vi "Text control 2 v0.4.vi"() -> ()   [LabVIEW 2016]
panel:
  out "Ion vs time":cluster{"Y data in":dbl[], "X data in":dbl[]}[](graph)
  out "Ig":dbl format="%.2e"
  out "Id":dbl format="%.2e"
  out "Is":dbl format="%.2e"
  out "I vs Vg":cluster{"Y data in":dbl[], "X data in":dbl[]}[](graph)
  in  "Suffix":string=".txt"
  in  "Prefix":string="-transfer-"
  in  "Panel Controls 2":T1={"Emergency Stop"=refnum, "TransGraph Max"=1e-05, "Text/Graph (text=false)"=TRUE, "TransGraph Min"=1e-11} {"TransGraph Min" format="%.2e"; "TransGraph Max" format="%.2e"}
  out "Currently running:":string="#output s 0 0 0 -0.008 0.008 0.002"
  in  "Lines left to run:":string
  in  "Standby":T2
  in  "Full Reset":bool
  in  "SMU4":cluster{"on/off":bool, "Voltage":dbl} {"Voltage" min=-100.0 max=100.0 format="%.2f"}
  in  "Source/Drain Range":u8(slide)=6 max=11 scale=0.0..11.0
  in  "Source/Drain\nRange mode":u16(ring) items=["Auto", "Limited", "Fixed"]
  in  "Gate Range":u8(slide)=6 max=11 scale=0.0..11.0
  in  "Gate Range\nmode":u16(ring) items=["Auto", "Limited", "Fixed"]
  in  "Gate":T3={"Gate Start"=0.0, "Gate Stop"=2.0, "Gate Step (linear only)"=1.0, "Gate Compliance"=0.0001, "Gate PComp"=0.0, "Range mode"=0, "Range"=6} {"Range" max=11 scale=0.0..11.0; "Range mode" items=["Auto", "Limited", "Fixed"]; "Gate PComp" format="%^.2e"; "Gate Compliance" format="%^.2e"; "Gate Step (linear only)" format="%^.4e"; "Gate Stop" format="%^.4e"; "Gate Start" format="%^.4e"}
  in  "Drain 2":T4={"Drain Start"=0.0, "Drain Stop"=2.0, "Drain Compliance"=0.0001, "Drain Step"=1.0, "Drain PComp"=0.0, "Range mode"=0, "Range"=6} {"Range" max=11 scale=0.0..11.0; "Range mode" items=["Auto", "Limited", "Fixed"]; "Drain PComp" format="%^.2e"; "Drain Step" format="%^.4e"; "Drain Compliance" format="%^.2e"; "Drain Stop" format="%^.4e"; "Drain Start" format="%^.4e"}
  in  "Timings 2":T5={"integration time"=0, "Short/Long integration time"=0.00064, "hold time (sec)"=0.0, "delay time (sec)"=0.0, "Step Time (0 disables)"=0.0, "sweep method"=0, "Pulse period"=0.005, "Base voltage"=0.0, "Pulse width"=0.0005} {"Pulse width" min=0.0005 max=0.1 step=0.0001 format="%.4f"; "Base voltage" format="%^.4e"; "Pulse period" min=0.005 max=1.0 step=0.0001 format="%.4f"; "sweep method" items=["Continuous", "Pulsed"]; "Step Time (0 disables)" format="%.2f"; "delay time (sec)" format="%.4f"; "hold time (sec)" format="%.4f"; "Short/Long integration time" format="%^.0e"; "integration time" scale=0.0..2.0}
  in  "Panel Controls":T6={"Emergency Stop"=refnum, "TransGraph Max"=1e-05, "Text/Graph (text=false)"=TRUE} {"TransGraph Max" format="%.2e"}
  in  "Interrupt run":bool
  in  "Drain: Compliance":dbl=0.001 format="%.8f"
  in  "Gate: Compliance":dbl=0.001 format="%.8f"
  out "Path":path=path "C:/users/rlp38/09Apr2009LTtesting/test2.txt"
  in  "hold time /s":dbl format="%.2f"
  in  "delay time /s":dbl format="%.2f"
  in  "integration time":u32(slide) max=2 step=1 scale=0.0..2.0
  in  "Integration time (short)":dbl=0.0019 min=8e-05 max=0.0019 step=8e-05 format="%^.0e"
  in  "Integration time (long)":dbl=0.32 min=0.04 max=2.0 step=0.02 format="%.2f"
  in  "Step delay /s":dbl format="%.2f"
  in  "Program":string="#pulsedstressV d 0.03 20 0 0.5 0.0827 5\n#\n#itime m\n#gaterangemode a\n#drainrangemode a\n#pulsed on 0.05 0 0.02\n#transfer d -10 40 1 5 40 35\n#transfer d -10 40 1 5 40 35\n#transfer d -10 40 1 5 40 35\n#output d 0 40 20 0 40 1\n#\n#\n#sample 1 0.008 221 6 0.003\n#samplei 400e-6 200 6 0.002 0.1\n#vsu2pulse -10 4\n#\n#stressV 0.016 0.03 2e-4 0.1e-3 11\n#stressI 220e-7 0.08 15\n#transfer s -1 1 0.5 -0.005 0.005 0.005\n#output s 0 0 0 -0.008 0.008 0.002\n"
  # "Syntax:\nitime [s|m|l]\ngaterangemode [a|l|f]\ndrainrangemode [a|l|f]\npulsed [on|off] PulsePeriod(sec) PulseBaseVoltage PulseONWidth(sec)\nstandby [on l off]\nwait NumMilliseconds\nwait-min NumMinutes\n# texthere = comment\ntransfer [s|d] VgStart VgStop VgStep VdStart VdStop VdStep\noutput [s|d] VgStart VgStop VgStep VdStart VdStop VdStep\nsample Vg Vd NumSamples Time(s) SampleInterval(s)\nsamplei Idg NumSamples Time(s) SampleInterval(s) VDGcompliance\n# if in doubt use SampleInterval(s) = 0.004\nstressV VG VD IGcompliance IDcompliance Duration(sec)\nstressI IDG VDGcompliance Duration(sec)\nvsu2pulse Bias Duration(s)\npulsedstressV [s|d] VEstop VgON VgOFF Period(s) PulseONwidth(s) Vd\nsample-fpp Vg Vd NumSamples Time\nresample-fpp Vg Vd\ntransfer-fpp [s|d] VgStart VgStop VgStep VdStart VdStop VdStep\noutput-fpp [s|d] VgStart VgStop VgStep VdStart VdStop VdStep"
  # "Original Filename (.txt is removed)-Prefix-ElapsedTime (in sec)-Suffix (must include .txt)"
  # "100 samples is approx 13s with medium integration"
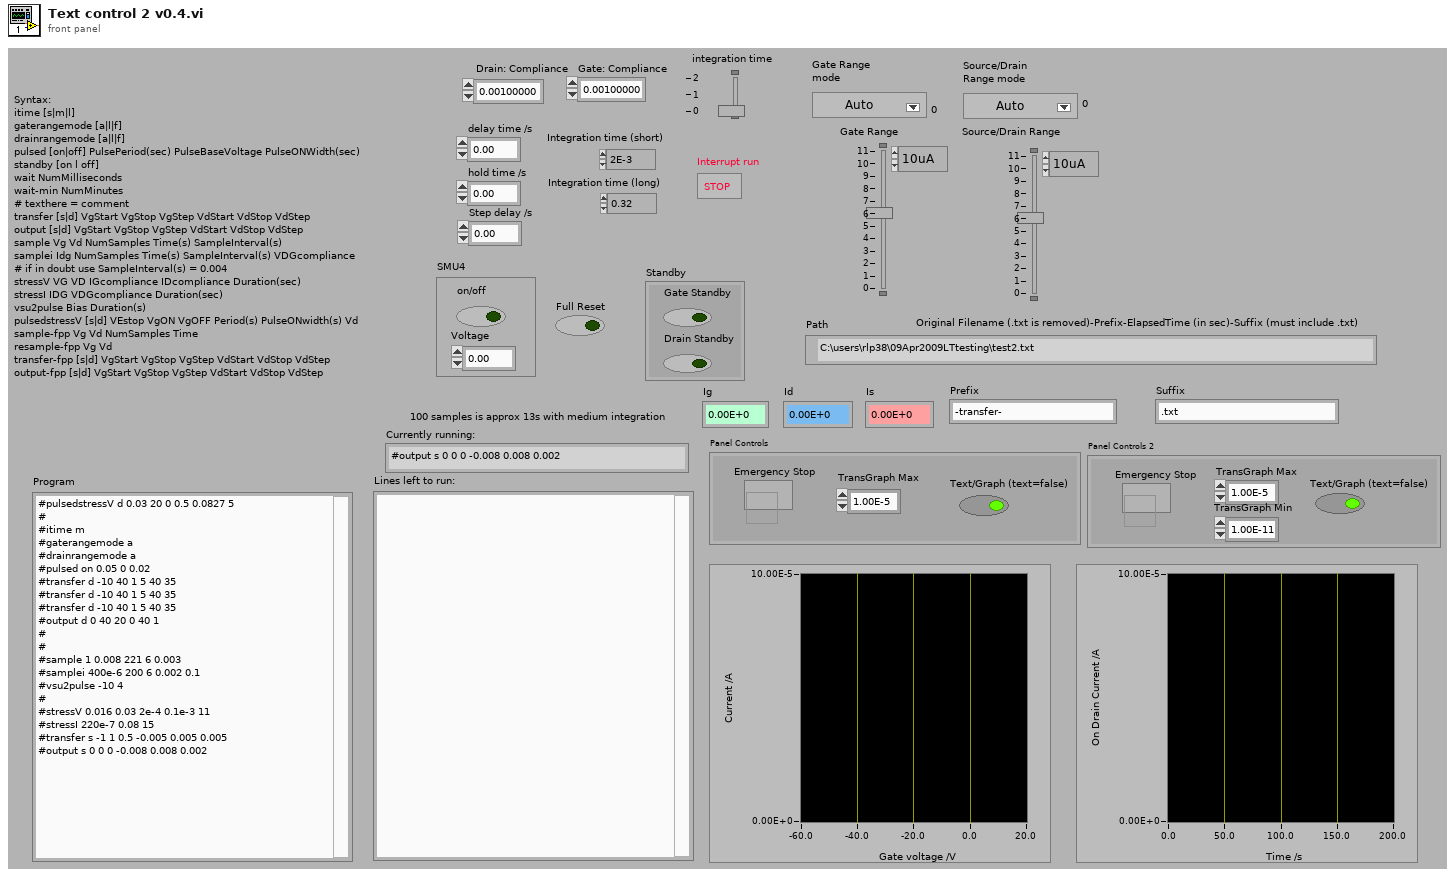
[diagram p1: front panel]
types:
  T1 = cluster{"Emergency Stop":refnum<vi>, "TransGraph Max":dbl, "Text/Graph (text=false)":bool, "TransGraph Min":dbl}
  T2 = cluster{"Gate Standby":bool, "Drain Standby":bool}
  T3 = cluster{"Gate Start":dbl, "Gate Stop":dbl, "Gate Step (linear only)":dbl, "Gate Compliance":dbl, "Gate PComp":dbl, "Range mode":u16, "Range":u8}
  T4 = cluster{"Drain Start":dbl, "Drain Stop":dbl, "Drain Compliance":dbl, "Drain Step":dbl, "Drain PComp":dbl, "Range mode":u16, "Range":u8}
  T5 = cluster{"integration time":u32, "Short/Long integration time":dbl, "hold time (sec)":dbl, "delay time (sec)":dbl, "Step Time (0 disables)":dbl, "sweep method":u16, "Pulse period":dbl, "Base voltage":dbl, "Pulse width":dbl}
  T6 = cluster{"Emergency Stop":refnum<vi>, "TransGraph Max":dbl, "Text/Graph (text=false)":bool}
  T7 = enum16{"open", "replace", "create", "open or create", "replace or create", "replace or create with confirmation"}
  T8 = cluster{"V2 Start":dbl, "V2 Step":dbl, "Number of points":i32}
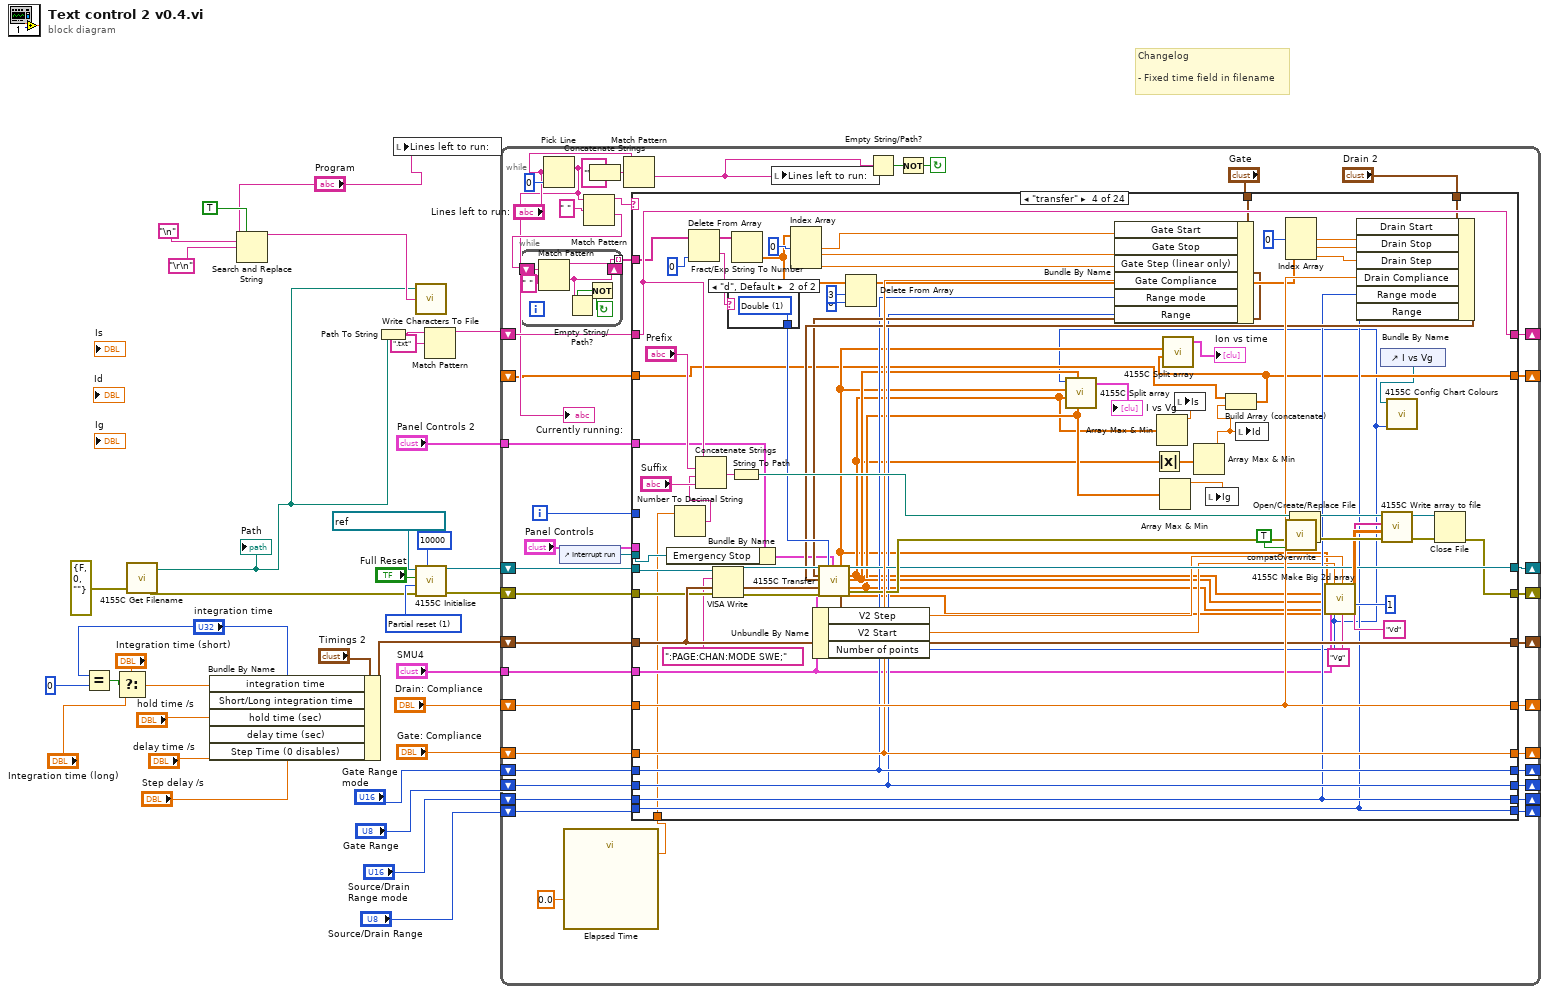
[diagram p0: block diagram]
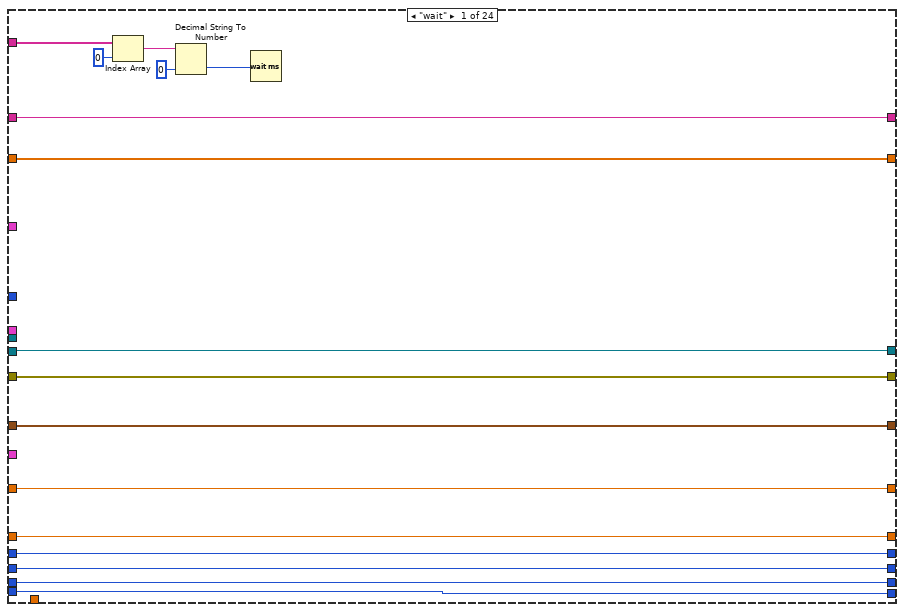
[diagram p2: hidden frame]
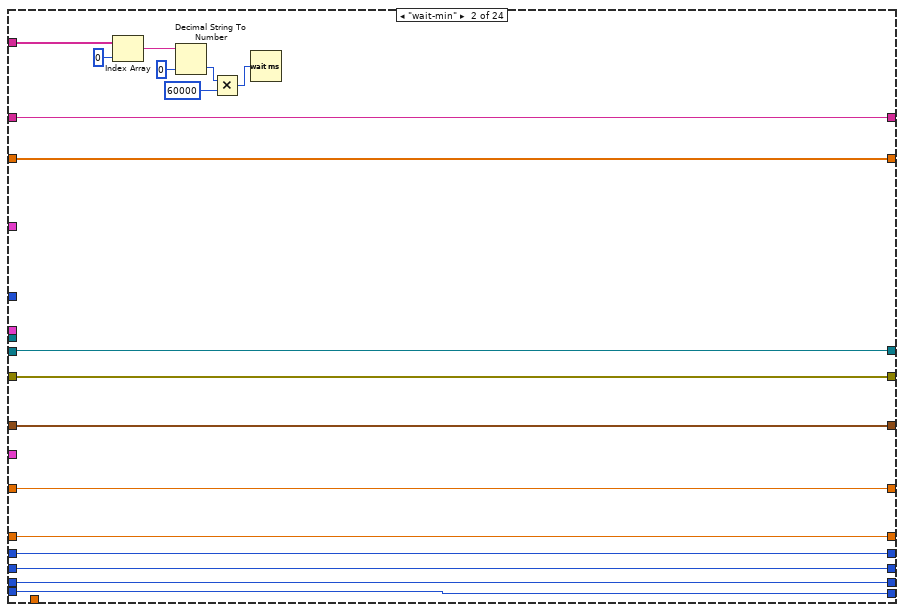
[diagram p3: hidden frame]
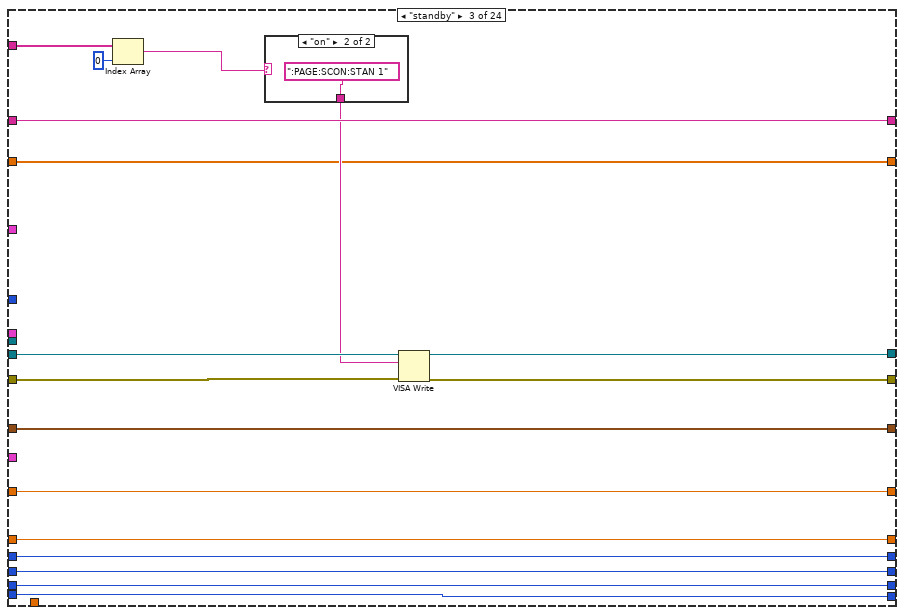
[diagram p4: hidden frame]
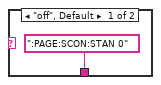
[diagram p5: hidden frame]
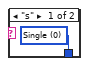
[diagram p6: hidden frame]
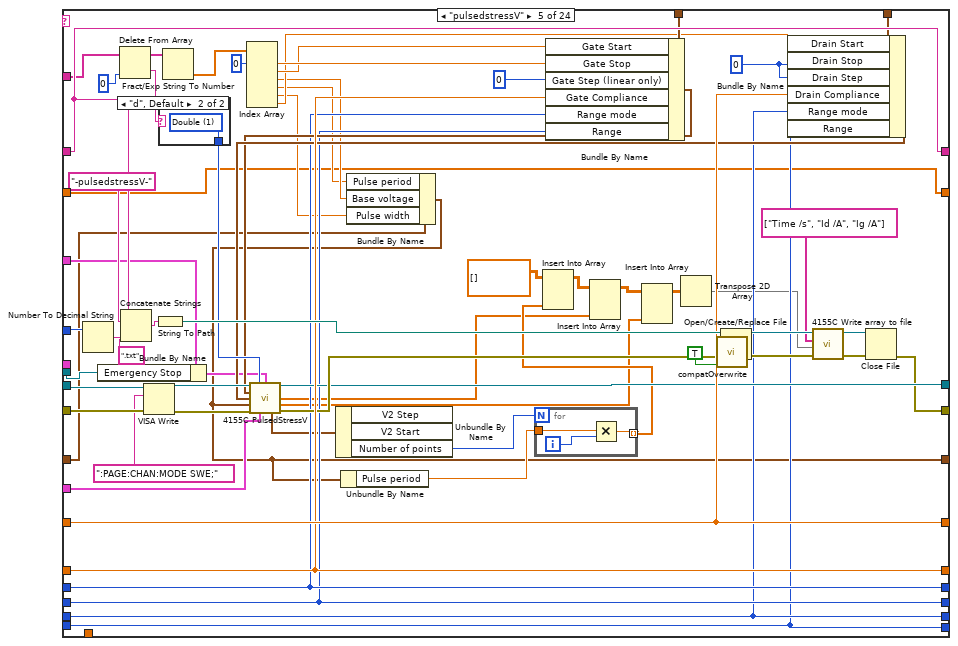
[diagram p7: hidden frame]
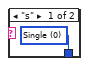
[diagram p8: hidden frame]
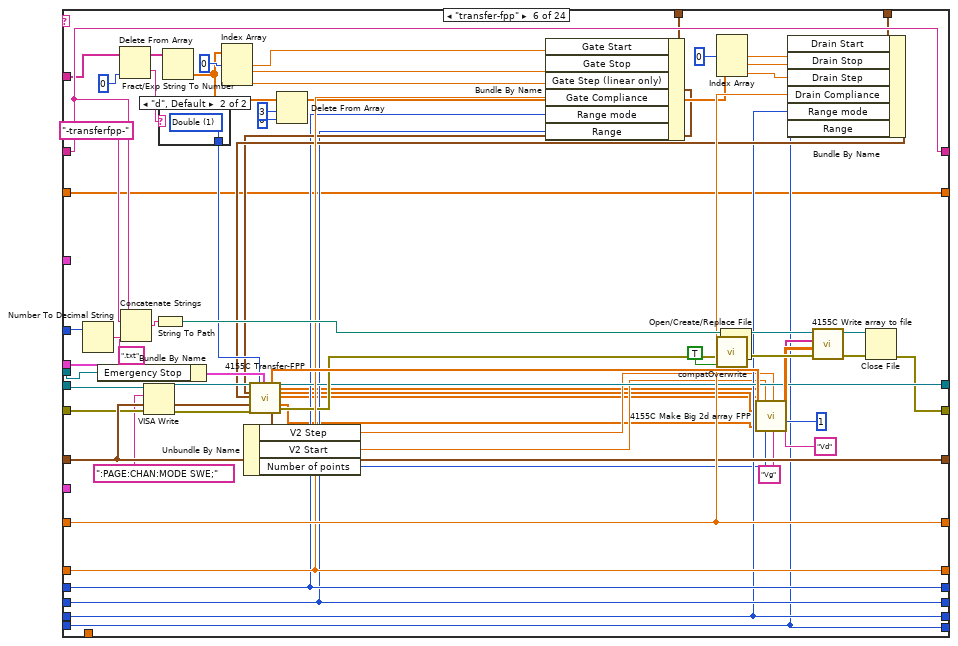
[diagram p9: hidden frame]
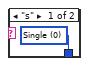
[diagram p10: hidden frame]
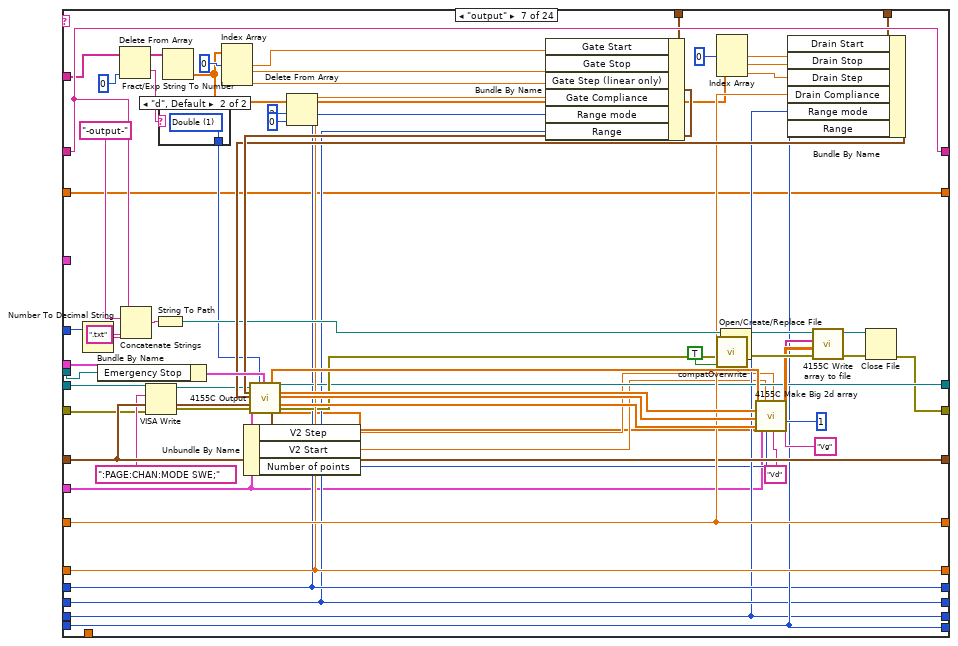
[diagram p11: hidden frame]
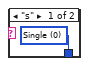
[diagram p12: hidden frame]
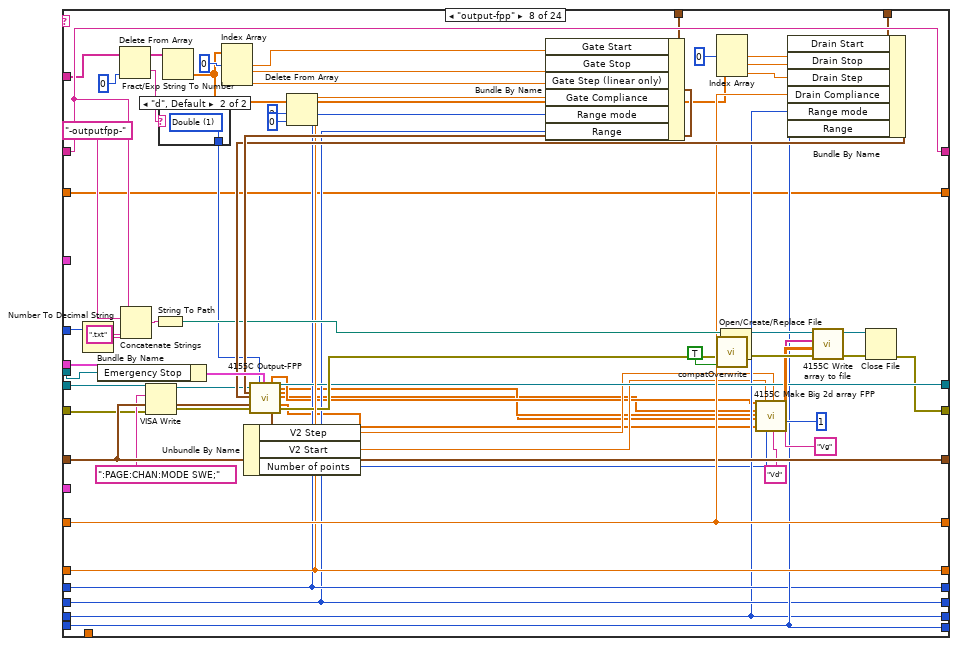
[diagram p13: hidden frame]
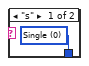
[diagram p14: hidden frame]
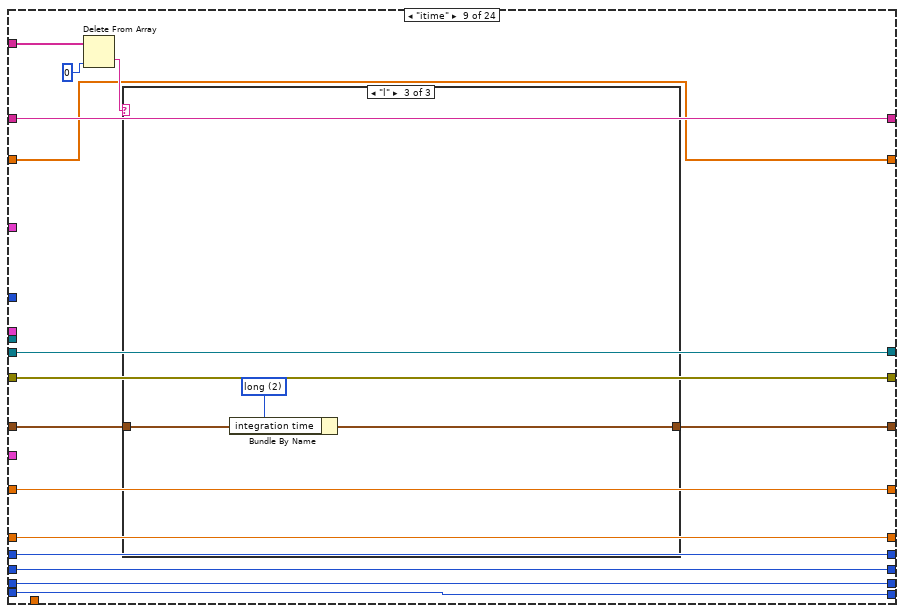
[diagram p15: hidden frame]
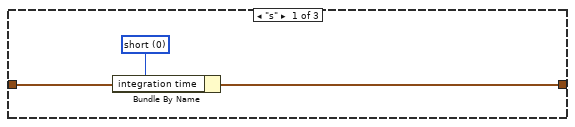
[diagram p16: hidden frame]
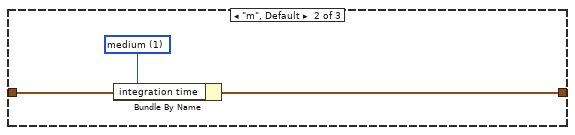
[diagram p17: hidden frame]
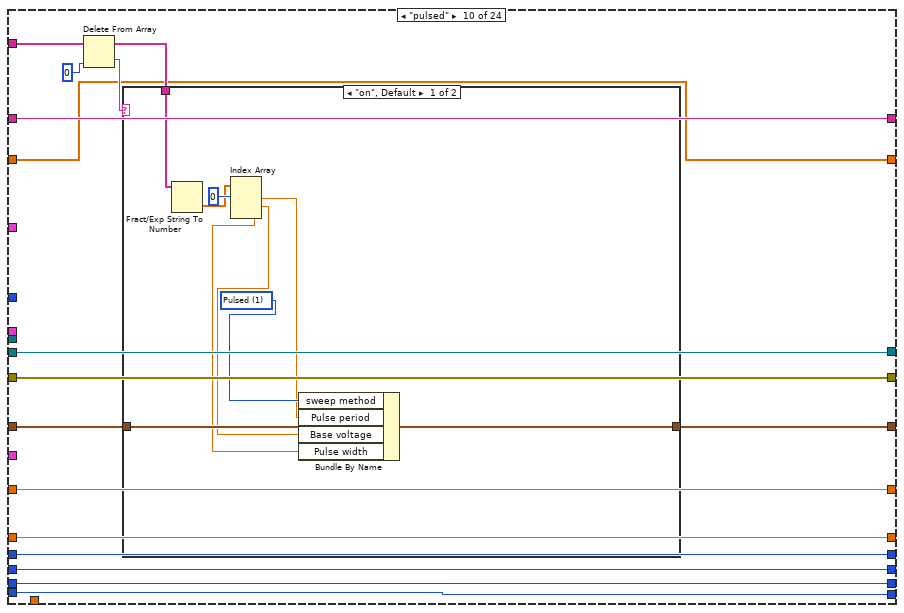
[diagram p18: hidden frame]
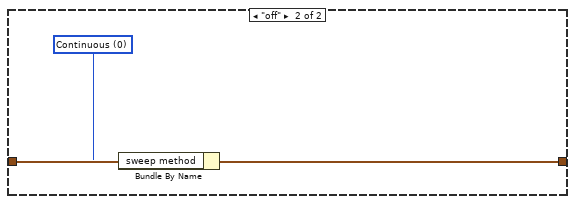
[diagram p19: hidden frame]
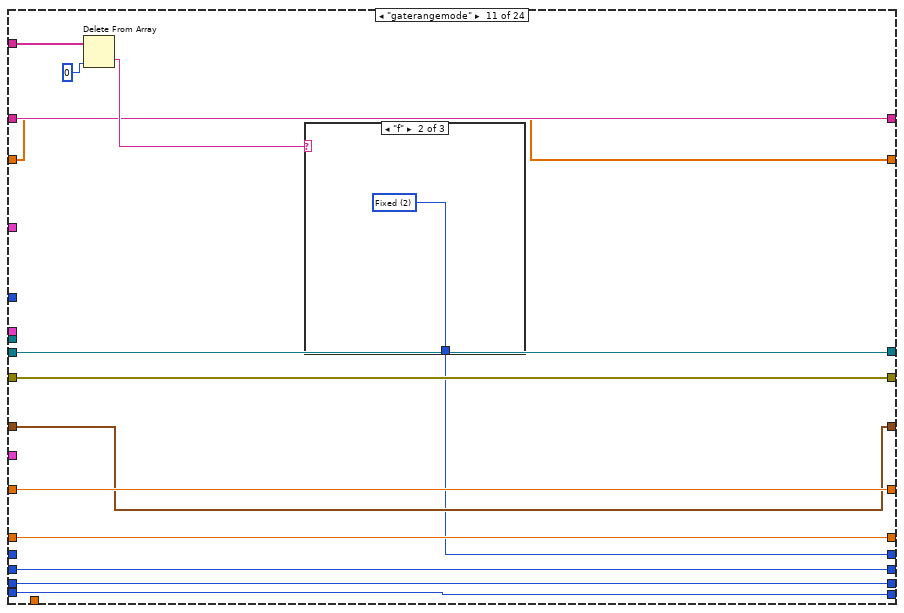
[diagram p20: hidden frame]
diagram:
  w27 = u16 1 items=["Reset All", "Partial reset"] ("Type of reset")
  # "Changelog\n\n- Fixed time field in filename"
  n1 = Equal?(x="integration time", y=u32 0) -> (x = y?=w31:bool)
  n2 = Select(t="Integration time (short)", s=w31, f="Integration time (long)") -> (s? t:f=w35:dbl)
  n3 = call <userlib>:"4155C Get Filename.vi"("error in (no error)"=errorcluster {"status"=FALSE, "code"=0, "source"=""}) -> ("error out"=w22:errorcluster, "path"=w6:path)  [unwired: 2 in, 1 out]
  "Path" <- w6
  n4 = Bundle By Name(cluster="Timings 2", "integration time"="integration time", "Short/Long integration time"=w35, "hold time (sec)"="hold time /s", "delay time (sec)"="delay time /s", "Step Time (0 disables)"="Step delay /s") -> (w19:T5)
  n5 = Search and Replace String(replace all?=TRUE ("replace all? (F)"), input string="Program", search string="\n", replace string="\r\n") -> (result string=w9:string)  [unwired: 4 in, 3 out]
  n6 = Path To String(path=w6) -> (string=w5:string)
  n7 = local write "Lines left to run:"("Program") -> ()
  n8 = call <vilib>:"Write Characters To File.vi"("character string"=w9, "file path (dialog if empty)"=w6) -> ()  [unwired: 3 in, 1 out]
  n9 = call <userlib>:"4155C Initialise.vi"("VISA resource name in"=refnum<visa-resource-name> "GPIB0::14::INSTR", "Reset"="Full Reset", "Type of reset"=w27, "error in (no error)"=w22, "VISA Timeout Value"=u32 10000) -> ("VISA Resource Name out"=w21:refnum<visa-resource-name>, "error out"=w20:errorcluster)
  n10 = Match Pattern(string=w5, regular expression=".txt") -> (before substring=w4:string)  [unwired: 1 in, 3 out]
  n11 = while {
    tunnel: "SMU4" -> [w45]
    shift-left: "Source/Drain Range" -> [w50]
    shift-right: [w46] -> _
    shift-left: "Source/Drain\nRange mode" -> [w51]
    shift-right: [w47] -> _
    shift-left: "Gate Range" -> [w52]
    shift-right: [w48] -> _
    shift-left: "Gate Range\nmode" -> [w53]
    shift-right: [w49] -> _
    shift-left: "Gate: Compliance" -> [w65]
    shift-right: [w59] -> _
    shift-left: "Drain: Compliance" -> [w66]
    shift-right: [w60] -> _
    shift-left: w19 -> [w67]
    shift-right: [w61] -> _
    shift-left: w20 -> [w68]
    shift-right: [w62] -> _
    shift-left: w21 -> [w69]
    shift-right: [w63] -> _
    shift-left: w4 -> [w70]
    shift-right: [w58] -> _
    tunnel: "Panel Controls 2" -> [w41]
    shift-right: [w40] -> _
    shift-left: _ -> [w39]
    i -> [w64]
    stop <- w78 continue-if-true
    n12 = Pick Line(multi-line string="Lines left to run:", line index=0) -> (output string=w42:string)  [unwired: 1 in]
    "Currently running:" <- w42
    n13 = control-ref of="Interrupt run"() -> (w57:refnum<vi>)
    n14 = call "Elapsed Time"("Set Start Time (s)"=0.0) -> ("Elapsed Time (s)"=w38:dbl)  [unwired: 11 in, 7 out]
    n15 = Match Pattern(string=w42, regular expression=" ") -> (before substring=w73:string, after substring=w72:string)  [unwired: 1 in, 2 out]
    n16 = while {
      tunnel: [w80] -> w71 mode=indexing
      shift-left: w72 -> [w82]
      shift-right: [w81] -> _
      stop <- w84 continue-if-true
      n17 = Match Pattern(string=w82, regular expression=" ") -> (before substring=w80:string, after substring=w81:string)  [unwired: 1 in, 2 out]
      n18 = Empty String/Path?(string/path=w81) -> (empty?=w85:bool)
      n19 = Not(x=w85) -> (.not. x?=w84:bool)
    }
    n20 = Concatenate Strings(w42, "\n" ("Substring")) -> (w76:string)
    n21 = Match Pattern(string="Lines left to run:", regular expression=w76) -> (after substring=w43:string)  [unwired: 1 in, 3 out]
    n22 = case shown="\"transfer\"" w73 {
      tunnel: w71 -> [w101 w119 w136 w196 w264 w331 w396 w469 w507 w532 w558 w582 w602 w615 _ _ w713 w772 _ w834 w876 w916 w984 w1044]
      tunnel: w70 -> [w96 w115 w134 w204 w271 w339 w404 w477 w496 w521 w550 w575 w596 w608 w626 w665 w691 w754 w785 w821 w863 w904 w978 w1040]
      tunnel: w69 -> [w95 w114 w125 w174 w255 w308 w372 w445 w497 w522 w551 w576 w597 w609 w631 w668 w720 w779 w789 w841 w883 w923 w991 w997]
      tunnel: w68 -> [w94 w113 w124 w173 w254 w307 w369 w442 w498 w523 w552 w577 w598 w610 w630 w637 w719 w778 w788 w840 w882 w922 w990 w996]
      tunnel: w67 -> [w93 w112 w133 w200 w229 w335 w400 w473 w506 w531 w549 w574 w595 w607 w629 w661 w682 w746 w794 w814 w856 w897 w977 w1039]
      tunnel: w66 -> [w92 w111 w132 w202 w269 w337 w402 w475 w505 w530 w557 w581 w601 w614 w628 w646 w718 w777 w797 w839 w881 w921 w989 w1049]
      tunnel: w65 -> [w91 w110 w131 w201 w268 w336 w401 w474 w504 w529 w556 w580 w600 w613 w627 w647 w692 w755 w796 w822 w864 w905 w979 w1041]
      tunnel: w64 -> [_ _ _ _ w272 w340 w405 w478 _ _ _ _ _ _ _ w663 w717 w776 _ w838 w880 w920 w988 w1048]
      tunnel: [w95 w114 w123 w198 w266 w333 w398 w471 w497 w522 w551 w576 w597 w609 w631 w668 w683 w727 w787 w815 w857 w898 w929 w999] -> w63
      tunnel: [w94 w113 w122 w197 w265 w332 w397 w470 w498 w523 w552 w577 w598 w610 w630 w636 w693 w728 w786 w823 w865 w906 w928 w998] -> w62
      tunnel: [w93 w112 w133 w200 w225 w335 w400 w473 w499 w524 w549 w574 w595 w607 w629 w661 w682 w746 w794 w814 w856 w897 w977 w1039] -> w61
      tunnel: [w92 w111 w132 w202 w269 w337 w402 w475 w505 w530 w557 w581 w601 w614 w628 w646 w718 w777 w797 w839 w881 w921 w989 w1049] -> w60
      tunnel: [w91 w110 w131 w201 w268 w336 w401 w474 w504 w529 w556 w580 w600 w613 w627 w647 w692 w755 w796 w822 w864 w905 w979 w1041] -> w59
      tunnel: [w96 w115 w134 w204 w271 w339 w404 w477 w496 w521 w550 w575 w596 w608 w626 w665 w691 w754 w785 w821 w863 w904 w978 w1040] -> w58
      tunnel: w57 -> [_ _ _ w207 w276 w345 w413 w482 _ _ _ _ _ _ _ _ w688 w751 _ w820 w862 w903 w949 w1015]
      tunnel: "Gate" -> [_ _ _ w183 w258 w318 w383 w456 _ _ _ _ _ _ _ _ _ _ _ _ _ _ _ _]
      tunnel: "Drain 2" -> [_ _ _ w182 w257 w317 w382 w455 _ _ _ _ _ _ _ _ _ _ _ _ _ _ _ _]
      tunnel: "Panel Controls" -> [_ _ _ _ _ w316 w381 w454 _ _ _ _ _ _ _ _ _ _ _ _ _ _ _ _]
      tunnel: w53 -> [w90 w109 w130 w167 w248 w301 w367 w440 w503 w528 _ w573 w594 w606 w625 w648 w678 w742 w790 w810 w852 w893 w973 w1035]
      tunnel: w52 -> [w89 w108 w129 w166 w247 w300 w366 w439 w502 w527 w555 _ w585 w612 w624 w649 w679 w743 w791 w811 w853 w894 w974 w1036]
      tunnel: w51 -> [w88 w107 w128 w165 w246 w299 w365 w438 w501 w526 w554 w579 w599 _ w623 w650 w680 w744 w792 w812 w854 w895 w975 w1037]
      tunnel: w50 -> [w87 w106 w127 w164 w245 w298 w368 w441 w500 w525 w553 w578 _ w611 w622 w651 w681 w745 w793 w813 w855 w896 w976 w1038]
      tunnel: [w90 w109 w130 w167 w248 w301 w367 w440 w503 w528 w548 w573 w594 w606 w625 w648 w678 w742 w790 w810 w852 w893 w973 w1035] -> w49
      tunnel: [w89 w108 w129 w166 w247 w300 w366 w439 w502 w527 w555 w565 w585 w612 w624 w649 w679 w743 w791 w811 w853 w894 w974 w1036] -> w48
      tunnel: [w88 w107 w128 w165 w246 w299 w365 w438 w501 w526 w554 w579 w599 w605 w623 w650 w680 w744 w792 w812 w854 w895 w975 w1037] -> w47
      tunnel: [w87 w106 w127 w164 w245 w298 w368 w441 w500 w525 w553 w578 w586 w611 w622 w651 w681 w745 w793 w813 w855 w896 w976 w1038] -> w46
      tunnel: w45 -> [_ _ _ w158 w241 _ w359 _ _ _ _ _ _ _ _ _ _ _ _ _ _ _ _ _]
      tunnel: w41 -> [_ _ _ w156 w240 _ _ _ _ _ _ _ _ _ _ _ _ _ _ _ _ _ _ _]
      tunnel: [w86 w102 w120 w145 w217 w287 w356 w426 w495 w519 w547 w564 w584 w604 w621 w632 w669 w725 w784 w798 w844 w886 w926 w992] -> w40
      tunnel: w39 -> [w86 w102 w120 w144 w217 w287 w356 w426 w495 w519 w547 w564 w584 w604 w621 w632 w669 w725 w784 w798 w844 w886 w926 w992]
      tunnel: w38 -> [_ _ _ w140 _ _ _ _ _ _ _ _ _ _ _ _ _ _ _ _ _ _ _ _]
      frame "wait" {
        n23 = Index Array(array=w101, index=0 ("Index")) -> (element=w99:string)
        n24 = Decimal String To Number(string=w99, default (0L)=u32 0) -> (number=w98:u32)  [unwired: 1 in, 1 out]
        n25 = Wait (ms)(milliseconds to wait=w98) -> ()  [unwired: 1 out]
      }
      frame "wait-min" {
        n26 = Index Array(array=w119, index=0 ("Index")) -> (element=w117:string)
        n27 = Decimal String To Number(string=w117, default (0L)=u32 0) -> (number=w105:u32)  [unwired: 1 in, 1 out]
        n28 = Multiply(x=w105, y=u32 60000) -> (x*y=w104:u32)
        n29 = Wait (ms)(milliseconds to wait=w104) -> ()  [unwired: 1 out]
      }
      frame "standby" {
        n30 = Index Array(array=w136, index=0 ("Index")) -> (element=w126:string)
        n31 = case shown="\"on\"" w126 {
          tunnel: [":PAGE:SCON:STAN 0" ":PAGE:SCON:STAN 1"] -> w121
          frame "off", Default {
          }
          frame "on" {
          }
        }
        n32 = VISA Write(VISA resource name=w125, write buffer=w121, error in (no error)=w124) -> (VISA resource name out=w123:refnum<visa-resource-name>, error out=w122:errorcluster)  [unwired: 1 out]
      }
      frame "transfer" {
        n33 = Bundle By Name(cluster=w156, "Emergency Stop"=w207) -> (w157:T1)
        n34 = Number To Decimal String(number=w140) -> (decimal integer string=w139:string)  [unwired: 1 in]
        n35 = Delete From Array(array=w196, index=0 ("Index")) -> (deleted portion=w194:string, array with subset deleted=w193:string[])  [unwired: 1 in]
        n36 = Concatenate Strings(w204, "Prefix", w139, "Suffix") -> (w206:string)
        n37 = VISA Write(VISA resource name=w174, write buffer=":PAGE:CHAN:MODE SWE;" ("write buffer (\"\")"), error in (no error)=w173) -> (VISA resource name out=w171:refnum<visa-resource-name>, error out=w172:errorcluster)  [unwired: 1 out]
        n38 = case shown="\"d\", Default" w194 {
          tunnel: [w215 w216] -> w192
          frame "s" {
            w215 = u16 0 items=["Single", "Double"] ("sweep mode")
          }
          frame "d", Default {
            w216 = u16 1 items=["Single", "Double"] ("sweep mode")
          }
        }
        n39 = String To Path(string=w206) -> (path=w203:path)
        n40 = Fract/Exp String To Number(string=w193) -> (number=w178:dbl[])  [unwired: 3 in, 1 out]
        n41 = Index Array(array=w178, index #1=0 ("Index")) -> (element #1=w191:dbl, element #2=w190:dbl, element #3=w189:dbl)  [unwired: 2 in]
        n42 = Delete From Array(array=w178, length=3 ("Length"), index=0 ("Index")) -> (array with subset deleted=w176:dbl[])  [unwired: 1 out]
        n43 = Bundle By Name(cluster=w183, "Gate Start"=w191, "Gate Stop"=w190, "Gate Step (linear only)"=w189, "Gate Compliance"=w201, "Range mode"=w167, "Range"=w166) -> (w168:T3)
        n44 = Index Array(array=w176, index #1=0 ("Index")) -> (element #1=w186:dbl, element #2=w185:dbl, element #3=w184:dbl)  [unwired: 2 in]
        n45 = call <vilib>:"compatOverwrite.vi"("overwrite (F)"=TRUE) -> ("overwrite?"=w155:T7)
        n46 = Bundle By Name(cluster=w182, "Drain Start"=w186, "Drain Stop"=w185, "Drain Step"=w184, "Drain Compliance"=w202, "Range mode"=w165, "Range"=w164) -> (w169:T4)
        n47 = call <userlib>:"4155C Transfer.vi"("VISA resource name in"=w171, "Gate"=w168, "Drain"=w169, "Timings"=w200, "error in (no error)"=w172, "SMU4"=w158, "sweep mode"=w192, "Panel Controls"=w157) -> ("VG"=w146:dbl[], "Outparams"=w162:T8, "VISA Resource Name out"=w198:refnum<visa-resource-name>, "IS"=w148:dbl[], "ID"=w153:dbl[], "IG"=w149:dbl[], "error out"=w199:errorcluster, "SMU4"=w159:dbl[])  [unwired: 12 in]
        n48 = Unbundle By Name(w162) -> ("V2 Step"=w161:dbl, "V2 Start"=w160:dbl, "Number of points"=w142:i32)
        n49 = call <userlib>:"4155C Split array.vi"("Number of VAR2 steps"=w142, "Y2 data in"=w153, "X data in"=w146, "Y1 data in"=w148, "Y3 data in"=w149) -> ("Array of clusters"=→"I vs Vg":cluster{"Y data in":dbl[], "X data in":dbl[]}[])  [unwired: 2 in, 1 out]
        n50 = Absolute Value(x=w148) -> (abs(x)=w152:dbl[])
        n51 = Array Max & Min(array=w148) -> (max value=w150:dbl)  [unwired: 3 out]
        n52 = Array Max & Min(array=w149) -> (max value=w151:dbl)  [unwired: 3 out]
        n53 = local write "Is"(w150) -> ()
        n54 = Array Max & Min(array=w152) -> (max value=w143:dbl)  [unwired: 3 out]
        n55 = local write "Ig"(w151) -> ()
        n56 = Build Array (concatenate)(w144, w143) -> (w145:dbl[])
        n57 = call <userlib>:"4155C Split array.vi"("X data in"=w146, "Y1 data in"=w145) -> ("Array of clusters"=→"Ion vs time":cluster{"Y data in":dbl[], "X data in":dbl[]}[])  [unwired: 5 in, 1 out]
        n58 = local write "Id"(w143) -> ()
        n59 = Open/Create/Replace File(file path (use dialog)=w203, error in=w199, operation (0:open)=w155) -> (refnum out=w212:refnum<file>, error out=w213:errorcluster)  [unwired: 3 in, 1 out]
        n60 = call <userlib>:"4155C Make Big 2d array.vi"("1D Var1"=w146, "1d IS"=w148, "1d ID"=w153, "1d IG"=w149, "1d SMU4"=w159, "SMU4"=w158, "VAR2 START"=w160, "Number of VAR2 steps"=w142, "VAR2 STEP"=w161, "VAR1 Name"="Vg", "Decimal places in header"=i8 1, "VAR2 Name"="Vd") -> ("Header array"=w208:string[], "Data array"=w209:dbl[][])  [unwired: 14 in]
        n61 = control-ref of="I vs Vg"() -> (w141:refnum<vi>)
        n62 = call <userlib>:"4155C Write array to file.vi"("Byte Stream File Refnum"=w212, "Header"=w208, "Data Array"=w209, "error in (no error)"=w213) -> ("dup refnum"=w210:refnum<file>, "error out"=w211:errorcluster)  [unwired: 1 in]
        n63 = call <userlib>:"4155C Config Chart Colours.vi"("Numeric"=w142, "XY Graph 2"=w141) -> ()  [unwired: 6 in]
        n64 = Close File(refnum=w210, error in=w211) -> (error out=w197:errorcluster)  [unwired: 1 out]
      }
      frame "pulsedstressV" {
        w223 = 0
        n65 = Number To Decimal String(number=w272) -> (decimal integer string=w273:string)  [unwired: 1 in]
        n66 = Bundle By Name(cluster=w240, "Emergency Stop"=w276) -> (w242:T1)
        n67 = Delete From Array(array=w264, index=0 ("Index")) -> (deleted portion=w262:string, array with subset deleted=w261:string[])  [unwired: 1 in]
        n68 = Concatenate Strings(w271, "-pulsedstressV-" ("Substring"), w273, ".txt" ("Substring")) -> (w275:string)
        n69 = VISA Write(VISA resource name=w255, write buffer=":PAGE:CHAN:MODE SWE;" ("write buffer (\"\")"), error in (no error)=w254) -> (VISA resource name out=w252:refnum<visa-resource-name>, error out=w253:errorcluster)  [unwired: 1 out]
        n70 = String To Path(string=w275) -> (path=w270:path)
        n71 = case shown="\"d\", Default" w262 {
          tunnel: [w285 w286] -> w260
          frame "s" {
            w285 = u16 0 items=["Single", "Double"] ("sweep mode")
          }
          frame "d", Default {
            w286 = u16 1 items=["Single", "Double"] ("sweep mode")
          }
        }
        n72 = Fract/Exp String To Number(string=w261) -> (number=w256:dbl[])  [unwired: 3 in, 1 out]
        n73 = Index Array(array=w256, index #1=0 ("Index")) -> (element #1=w232:dbl, element #2=w231:dbl, element #3=w228:dbl, element #4=w227:dbl, element #5=w226:dbl, element #6=w230:dbl)  [unwired: 5 in]
        n74 = Bundle By Name(cluster=w229, "Pulse period"=w227, "Base voltage"=w228, "Pulse width"=w226) -> (w225:T5)
        n75 = Unbundle By Name(w225) -> ("Pulse period"=w233:dbl)
        n76 = Bundle By Name(cluster=w258, "Gate Start"=w231, "Gate Stop"=w232, "Gate Step (linear only)"=0, "Gate Compliance"=w268, "Range mode"=w248, "Range"=w247) -> (w249:T3)
        n77 = call <vilib>:"compatOverwrite.vi"("overwrite (F)"=TRUE) -> ("overwrite?"=w218:T7)
        n78 = Bundle By Name(cluster=w257, "Drain Start"=w230, "Drain Stop"=w223, "Drain Step"=w223, "Drain Compliance"=w269, "Range mode"=w246, "Range"=w245) -> (w250:T4)
        n79 = call <userlib>:"4155C PulsedStressV.vi"("VISA resource name in"=w252, "sweep mode"=w260, "Panel Controls"=w242, "Gate"=w249, "Drain"=w250, "Timings"=w225, "error in (no error)"=w253, "SMU4"=w241) -> ("VISA Resource Name out"=w266:refnum<visa-resource-name>, "ID"=w221:dbl[], "IG"=w219:dbl[], "Outparams"=w243:T8, "error out"=w267:errorcluster)  [unwired: 3 in]
        n80 = Unbundle By Name(w243) -> ("Number of points"=w220:i32)  [unwired: 2 out]
        n81 = for {
          N: w220 -> [_]
          tunnel: [w282] -> w222 mode=indexing
          tunnel: w233 -> [w284]
          i -> [w283]
          n82 = Multiply(x=w284, y=w283) -> (x*y=w282:dbl)
        }
        n83 = Insert Into Array(array=dbl[][] [] ("Input Array"), new element=w222) -> (w234:dbl[][])  [unwired: 2 in]
        n84 = Insert Into Array(array=w234, new element=w221) -> (w239:dbl[][])  [unwired: 2 in]
        n85 = Insert Into Array(array=w239, new element=w219) -> (w238:dbl[][])  [unwired: 2 in]
        n86 = Transpose 2D Array(2D array=w238) -> (transposed array=w237:dbl[][])
        n87 = Open/Create/Replace File(file path (use dialog)=w270, error in=w267, operation (0:open)=w218) -> (refnum out=w279:refnum<file>, error out=w280:errorcluster)  [unwired: 3 in, 1 out]
        n88 = call <userlib>:"4155C Write array to file.vi"("Byte Stream File Refnum"=w279, "Header"=string[] ["Time /s", "Id /A", "Ig /A"], "Data Array"=w237, "error in (no error)"=w280) -> ("dup refnum"=w277:refnum<file>, "error out"=w278:errorcluster)  [unwired: 1 in]
        n89 = Close File(refnum=w277, error in=w278) -> (error out=w265:errorcluster)  [unwired: 1 out]
      }
      frame "transfer-fpp" {
        n90 = Number To Decimal String(number=w340) -> (decimal integer string=w341:string)  [unwired: 1 in]
        n91 = Bundle By Name(cluster=w316, "Emergency Stop"=w345) -> (w353:T6)
        n92 = Delete From Array(array=w331, index=0 ("Index")) -> (deleted portion=w329:string, array with subset deleted=w328:string[])  [unwired: 1 in]
        n93 = Concatenate Strings(w339, "-transferfpp-" ("Substring"), w341, ".txt" ("Substring")) -> (w343:string)
        n94 = VISA Write(VISA resource name=w308, write buffer=":PAGE:CHAN:MODE SWE;" ("write buffer (\"\")"), error in (no error)=w307) -> (VISA resource name out=w305:refnum<visa-resource-name>, error out=w306:errorcluster)  [unwired: 1 out]
        n95 = String To Path(string=w343) -> (path=w338:path)
        n96 = case shown="\"d\", Default" w329 {
          tunnel: [w354 w355] -> w327
          frame "s" {
            w354 = u16 0 items=["Single", "Double"] ("sweep mode")
          }
          frame "d", Default {
            w355 = u16 1 items=["Single", "Double"] ("sweep mode")
          }
        }
        n97 = Fract/Exp String To Number(string=w328) -> (number=w312:dbl[])  [unwired: 3 in, 1 out]
        n98 = Index Array(array=w312, index #1=0 ("Index")) -> (element #1=w326:dbl, element #2=w325:dbl, element #3=w324:dbl)  [unwired: 2 in]
        n99 = Delete From Array(array=w312, length=3 ("Length"), index=0 ("Index")) -> (array with subset deleted=w310:dbl[])  [unwired: 1 out]
        n100 = Bundle By Name(cluster=w318, "Gate Start"=w326, "Gate Stop"=w325, "Gate Step (linear only)"=w324, "Gate Compliance"=w336, "Range mode"=w301, "Range"=w300) -> (w302:T3)
        n101 = Index Array(array=w310, index #1=0 ("Index")) -> (element #1=w321:dbl, element #2=w320:dbl, element #3=w319:dbl)  [unwired: 2 in]
        n102 = call <vilib>:"compatOverwrite.vi"("overwrite (F)"=TRUE) -> ("overwrite?"=w288:T7)
        n103 = Bundle By Name(cluster=w317, "Drain Start"=w321, "Drain Stop"=w320, "Drain Step"=w319, "Drain Compliance"=w337, "Range mode"=w299, "Range"=w298) -> (w303:T4)
        n104 = call <userlib>:"4155C Transfer-FPP.vi"("VISA resource name in"=w305, "Gate"=w302, "Drain"=w303, "Timings"=w335, "error in (no error)"=w306, "sweep mode"=w327, "Panel Controls"=w353) -> ("VG"=w344:dbl[], "Outparams"=w296:T8, "VISA Resource Name out"=w333:refnum<visa-resource-name>, "Vprobe2"=w292:dbl[], "ID"=w291:dbl[], "IG"=w290:dbl[], "Vprobe1"=w289:dbl[], "error out"=w334:errorcluster)  [unwired: 13 in]
        n105 = Unbundle By Name(w296) -> ("V2 Step"=w295:dbl, "V2 Start"=w294:dbl, "Number of points"=w293:i32)
        n106 = Open/Create/Replace File(file path (use dialog)=w338, error in=w334, operation (0:open)=w288) -> (refnum out=w350:refnum<file>, error out=w351:errorcluster)  [unwired: 3 in, 1 out]
        n107 = call <userlib>:"4155C Make Big 2d array FPP.vi"("1D Var1"=w344, "1d ID"=w291, "1d Vp2"=w292, "1d IG"=w290, "1d Vp1"=w289, "VAR2 START"=w294, "Number of VAR2 steps"=w293, "VAR2 STEP"=w295, "VAR1 Name"="Vg", "Decimal places in header"=i8 1, "VAR2 Name"="Vd") -> ("Header array"=w346:string[], "Data array"=w347:dbl[][])  [unwired: 15 in]
        n108 = call <userlib>:"4155C Write array to file.vi"("Byte Stream File Refnum"=w350, "Header"=w346, "Data Array"=w347, "error in (no error)"=w351) -> ("dup refnum"=w348:refnum<file>, "error out"=w349:errorcluster)  [unwired: 1 in]
        n109 = Close File(refnum=w348, error in=w349) -> (error out=w332:errorcluster)  [unwired: 1 out]
      }
      frame "output" {
        n110 = Number To Decimal String(number=w405) -> (decimal integer string=w406:string)  [unwired: 1 in]
        n111 = Bundle By Name(cluster=w381, "Emergency Stop"=w413) -> (w423:T6)
        n112 = Delete From Array(array=w396, index=0 ("Index")) -> (deleted portion=w394:string, array with subset deleted=w393:string[])  [unwired: 1 in]
        n113 = Concatenate Strings(w404, "-output-" ("Substring"), w406, ".txt" ("Substring")) -> (w408:string)
        n114 = VISA Write(VISA resource name=w372, write buffer=":PAGE:CHAN:MODE SWE;" ("write buffer (\"\")"), error in (no error)=w369) -> (VISA resource name out=w371:refnum<visa-resource-name>, error out=w370:errorcluster)  [unwired: 1 out]
        n115 = String To Path(string=w408) -> (path=w403:path)
        n116 = case shown="\"d\", Default" w394 {
          tunnel: [w424 w425] -> w392
          frame "s" {
            w424 = u16 0 items=["Single", "Double"] ("sweep mode")
          }
          frame "d", Default {
            w425 = u16 1 items=["Single", "Double"] ("sweep mode")
          }
        }
        n117 = Fract/Exp String To Number(string=w393) -> (number=w375:dbl[])  [unwired: 3 in, 1 out]
        n118 = Index Array(array=w375, index #1=0 ("Index")) -> (element #1=w391:dbl, element #2=w390:dbl, element #3=w389:dbl)  [unwired: 2 in]
        n119 = Delete From Array(array=w375, length=3 ("Length"), index=0 ("Index")) -> (array with subset deleted=w374:dbl[])  [unwired: 1 out]
        n120 = Bundle By Name(cluster=w383, "Gate Start"=w391, "Gate Stop"=w390, "Gate Step (linear only)"=w389, "Gate Compliance"=w401, "Range mode"=w367, "Range"=w366) -> (w422:T3)
        n121 = Index Array(array=w374, index #1=0 ("Index")) -> (element #1=w386:dbl, element #2=w385:dbl, element #3=w384:dbl)  [unwired: 2 in]
        n122 = call <vilib>:"compatOverwrite.vi"("overwrite (F)"=TRUE) -> ("overwrite?"=w357:T7)
        n123 = Bundle By Name(cluster=w382, "Drain Start"=w386, "Drain Stop"=w385, "Drain Step"=w384, "Drain Compliance"=w402, "Range mode"=w365, "Range"=w368) -> (w421:T4)
        n124 = call <userlib>:"4155C Output.vi"("VISA resource name in"=w371, "Gate"=w422, "Drain"=w421, "Timings"=w400, "error in (no error)"=w370, "SMU4"=w359, "sweep mode"=w392, "Panel controls"=w423) -> ("VD"=w409:dbl[], "Outparams"=w362:T8, "VISA Resource Name out"=w398:refnum<visa-resource-name>, "IS"=w412:dbl[], "ID"=w411:dbl[], "IG"=w410:dbl[], "error out"=w399:errorcluster, "SMU4"=w358:dbl[])  [unwired: 12 in]
        n125 = Unbundle By Name(w362) -> ("V2 Step"=w363:dbl, "V2 Start"=w361:dbl, "Number of points"=w360:i32)
        n126 = Open/Create/Replace File(file path (use dialog)=w403, error in=w399, operation (0:open)=w357) -> (refnum out=w418:refnum<file>, error out=w419:errorcluster)  [unwired: 3 in, 1 out]
        n127 = call <userlib>:"4155C Make Big 2d array.vi"("1D Var1"=w409, "1d IS"=w412, "1d ID"=w411, "1d IG"=w410, "1d SMU4"=w358, "SMU4"=w359, "VAR2 START"=w361, "Number of VAR2 steps"=w360, "VAR2 STEP"=w363, "VAR1 Name"="Vd", "Decimal places in header"=i8 1, "VAR2 Name"="Vg") -> ("Header array"=w414:string[], "Data array"=w415:dbl[][])  [unwired: 14 in]
        n128 = call <userlib>:"4155C Write array to file.vi"("Byte Stream File Refnum"=w418, "Header"=w414, "Data Array"=w415, "error in (no error)"=w419) -> ("dup refnum"=w416:refnum<file>, "error out"=w417:errorcluster)  [unwired: 1 in]
        n129 = Close File(refnum=w416, error in=w417) -> (error out=w397:errorcluster)  [unwired: 1 out]
      }
      frame "output-fpp" {
        n130 = Number To Decimal String(number=w478) -> (decimal integer string=w479:string)  [unwired: 1 in]
        n131 = Bundle By Name(cluster=w454, "Emergency Stop"=w482) -> (w492:T6)
        n132 = Delete From Array(array=w469, index=0 ("Index")) -> (deleted portion=w467:string, array with subset deleted=w466:string[])  [unwired: 1 in]
        n133 = Concatenate Strings(w477, "-outputfpp-" ("Substring"), w479, ".txt" ("Substring")) -> (w481:string)
        n134 = VISA Write(VISA resource name=w445, write buffer=":PAGE:CHAN:MODE SWE;" ("write buffer (\"\")"), error in (no error)=w442) -> (VISA resource name out=w444:refnum<visa-resource-name>, error out=w443:errorcluster)  [unwired: 1 out]
        n135 = String To Path(string=w481) -> (path=w476:path)
        n136 = case shown="\"d\", Default" w467 {
          tunnel: [w493 w494] -> w465
          frame "s" {
            w493 = u16 0 items=["Single", "Double"] ("sweep mode")
          }
          frame "d", Default {
            w494 = u16 1 items=["Single", "Double"] ("sweep mode")
          }
        }
        n137 = Fract/Exp String To Number(string=w466) -> (number=w448:dbl[])  [unwired: 3 in, 1 out]
        n138 = Index Array(array=w448, index #1=0 ("Index")) -> (element #1=w464:dbl, element #2=w463:dbl, element #3=w462:dbl)  [unwired: 2 in]
        n139 = Delete From Array(array=w448, length=3 ("Length"), index=0 ("Index")) -> (array with subset deleted=w447:dbl[])  [unwired: 1 out]
        n140 = Bundle By Name(cluster=w456, "Gate Start"=w464, "Gate Stop"=w463, "Gate Step (linear only)"=w462, "Gate Compliance"=w474, "Range mode"=w440, "Range"=w439) -> (w491:T3)
        n141 = Index Array(array=w447, index #1=0 ("Index")) -> (element #1=w459:dbl, element #2=w458:dbl, element #3=w457:dbl)  [unwired: 2 in]
        n142 = call <vilib>:"compatOverwrite.vi"("overwrite (F)"=TRUE) -> ("overwrite?"=w427:T7)
        n143 = Bundle By Name(cluster=w455, "Drain Start"=w459, "Drain Stop"=w458, "Drain Step"=w457, "Drain Compliance"=w475, "Range mode"=w438, "Range"=w441) -> (w490:T4)
        n144 = call <userlib>:"4155C Output-FPP.vi"("VISA resource name in"=w444, "Gate"=w491, "Drain"=w490, "Timings"=w473, "error in (no error)"=w443, "sweep mode"=w465, "Panel controls"=w492) -> ("VD"=w432:dbl[], "Outparams"=w435:T8, "VISA Resource Name out"=w471:refnum<visa-resource-name>, "Vprobe2"=w431:dbl[], "ID"=w430:dbl[], "IG"=w429:dbl[], "Vprobe1"=w428:dbl[], "error out"=w472:errorcluster)  [unwired: 13 in]
        n145 = Unbundle By Name(w435) -> ("V2 Step"=w436:dbl, "V2 Start"=w434:dbl, "Number of points"=w433:i32)
        n146 = Open/Create/Replace File(file path (use dialog)=w476, error in=w472, operation (0:open)=w427) -> (refnum out=w487:refnum<file>, error out=w488:errorcluster)  [unwired: 3 in, 1 out]
        n147 = call <userlib>:"4155C Make Big 2d array FPP.vi"("1D Var1"=w432, "1d ID"=w430, "1d Vp2"=w431, "1d IG"=w429, "1d Vp1"=w428, "VAR2 START"=w434, "Number of VAR2 steps"=w433, "VAR2 STEP"=w436, "VAR1 Name"="Vd", "Decimal places in header"=i8 1, "VAR2 Name"="Vg") -> ("Header array"=w483:string[], "Data array"=w484:dbl[][])  [unwired: 15 in]
        n148 = call <userlib>:"4155C Write array to file.vi"("Byte Stream File Refnum"=w487, "Header"=w483, "Data Array"=w484, "error in (no error)"=w488) -> ("dup refnum"=w485:refnum<file>, "error out"=w486:errorcluster)  [unwired: 1 in]
        n149 = Close File(refnum=w485, error in=w486) -> (error out=w470:errorcluster)  [unwired: 1 out]
      }
      frame "itime" {
        n150 = Delete From Array(array=w507, index=0 ("Index")) -> (deleted portion=w508:string)  [unwired: 1 in, 1 out]
        n151 = case shown="\"l\"" w508 {
          tunnel: w506 -> [w512 w514 w517]
          tunnel: [w511 w513 w516] -> w499
          frame "s" {
            w510 = u32 0 items=["short  ", "medium  ", "long  "] ("integration time 2")
            n152 = Bundle By Name(cluster=w512, "integration time"=w510) -> (w511:T5)
          }
          frame "m", Default {
            w515 = u32 1 items=["short  ", "medium  ", "long  "] ("integration time 2")
            n153 = Bundle By Name(cluster=w514, "integration time"=w515) -> (w513:T5)
          }
          frame "l" {
            w518 = u32 2 items=["short  ", "medium  ", "long  "] ("integration time 2")
            n154 = Bundle By Name(cluster=w517, "integration time"=w518) -> (w516:T5)
          }
        }
      }
      frame "pulsed" {
        n155 = Delete From Array(array=w532, index=0 ("Index")) -> (deleted portion=w533:string, array with subset deleted=w520:string[])  [unwired: 1 in]
        n156 = case shown="\"on\", Default" w533 {
          tunnel: w531 -> [w543 w546]
          tunnel: [w542 w545] -> w524
          tunnel: w520 -> [w540 _]
          frame "on", Default {
            w541 = u16 1 items=["Continuous", "Pulsed"] ("sweep method")
            n157 = Fract/Exp String To Number(string=w540) -> (number=w538:dbl[])  [unwired: 3 in, 1 out]
            n158 = Index Array(array=w538, index #1=0 ("Index")) -> (element #1=w537:dbl, element #2=w536:dbl, element #3=w535:dbl)  [unwired: 2 in]
            n159 = Bundle By Name(cluster=w543, "sweep method"=w541, "Pulse period"=w537, "Base voltage"=w536, "Pulse width"=w535) -> (w542:T5)
          }
          frame "off" {
            w544 = u16 0 items=["Continuous", "Pulsed"] ("sweep method")
            n160 = Bundle By Name(cluster=w546, "sweep method"=w544) -> (w545:T5)
          }
        }
      }
      frame "gaterangemode" {
        n161 = Delete From Array(array=w558, index=0 ("Index")) -> (deleted portion=w559:string)  [unwired: 1 in, 1 out]
        n162 = case shown="\"f\"" w559 {
          tunnel: [w561 w562 w563] -> w548
          frame "a", Default {
            w561 = u16 0 items=["Auto", "Limited", "Fixed"] ("Gate Range\nmode 2")
          }
          frame "f" {
            w562 = u16 2 items=["Auto", "Limited", "Fixed"] ("Gate Range\nmode 2")
          }
          frame "l" {
            w563 = u16 1 items=["Auto", "Limited", "Fixed"] ("Gate Range\nmode 2")
          }
        }
      }
      frame "gaterange" {
        (unwired) u8 11 items=["10fA  ", "100fA  ", "1nA  ", "10nA", "100nA", "1uA", "10uA", "100uA", "1mA", "10mA", "100mA", "1A"] ("Gate Range 2")
        n163 = Delete From Array(array=w582, index=0 ("Index")) -> (deleted portion=w572:string)  [unwired: 1 in, 1 out]
        n164 = Scan Value(string=w572, format string="") -> (value=w570:dbl)  [unwired: 1 in, 1 out]
        n165 = Logarithm Base 10(1:w570) -> (0:w569:dbl)
        n166 = Round To Nearest(number=w569) -> (nearest integer value=w568:dbl)
        n167 = Add(x=w568, y=11.0) -> (x+y=w566:dbl)
        n168 = To Unsigned Byte Integer(number=w566) -> (unsigned 8bit integer=w565:u8)
      }
      frame "drainrange" {
        (unwired) u8 11 items=["10fA  ", "100fA  ", "1nA  ", "10nA", "100nA", "1uA", "10uA", "100uA", "1mA", "10mA", "100mA", "1A"] ("Gate Range 2")
        n169 = Delete From Array(array=w602, index=0 ("Index")) -> (deleted portion=w593:string)  [unwired: 1 in, 1 out]
        n170 = Scan Value(string=w593, format string="") -> (value=w591:dbl)  [unwired: 1 in, 1 out]
        n171 = Logarithm Base 10(1:w591) -> (0:w590:dbl)
        n172 = Round To Nearest(number=w590) -> (nearest integer value=w589:dbl)
        n173 = Add(x=w589, y=11.0) -> (x+y=w587:dbl)
        n174 = To Unsigned Byte Integer(number=w587) -> (unsigned 8bit integer=w586:u8)
      }
      frame "drainrangemode" {
        n175 = Delete From Array(array=w615, index=0 ("Index")) -> (deleted portion=w616:string)  [unwired: 1 in, 1 out]
        n176 = case shown="\"f\"" w616 {
          tunnel: [w618 w619 w620] -> w605
          frame "a", Default {
            w618 = u16 0 items=["Auto", "Limited", "Fixed"] ("Gate Range\nmode 2")
          }
          frame "f" {
            w619 = u16 2 items=["Auto", "Limited", "Fixed"] ("Gate Range\nmode 2")
          }
          frame "l" {
            w620 = u16 1 items=["Auto", "Limited", "Fixed"] ("Gate Range\nmode 2")
          }
        }
      }
      frame "Error", Default {
      }
      frame "logfile" {
        n177 = Number To Decimal String(number=w663) -> (decimal integer string=w667:string)  [unwired: 1 in]
        n178 = Concatenate Strings(w665, "logfile" ("Substring"), w667, ".txt" ("Substring")) -> (w662:string)
        n179 = String To Path(string=w662) -> (path=w635:path)
        n180 = Unbundle(w661) -> ("integration time"=w660:u32, "Short/Long integration time"=w659:dbl, "hold time (sec)"=w658:dbl, "delay time (sec)"=w657:dbl, "Step Time (0 disables)"=w656:dbl, "sweep method"=w655:u16, "Pulse period"=w654:dbl, "Base voltage"=w653:dbl, "Pulse width"=w652:dbl)
        n181 = Build Array(w660, w659, w658, w657, w656, w655, w654, w653, w652, w646, w647, w648, w649, w650, w651) -> (w639:dbl[])
        n182 = Insert Into Array(array=dbl[][] [] ("Input Array"), new element=w639) -> (w638:dbl[][])  [unwired: 2 in]
        n183 = call <vilib>:"compatOverwrite.vi"("overwrite (F)"=TRUE) -> ("overwrite?"=w633:T7)
        n184 = Open/Create/Replace File(file path (use dialog)=w635, error in=w637, operation (0:open)=w633) -> (refnum out=w643:refnum<file>, error out=w642:errorcluster)  [unwired: 3 in, 1 out]
        n185 = call <userlib>:"4155C Write array to file.vi"("Byte Stream File Refnum"=w643, "Header"=string[] ["Int Time", "Short/Long Itime", "Hold time", "Delay time", "Step time", "Sweep method", "Pulse period", "Base Voltage", "Pulse width", "Drain compliance", "Gate compliance", "Gate range mode", "Gate range", "S/D range mode", "S/D range"], "Data Array"=w638, "error in (no error)"=w642) -> ("dup refnum"=w645:refnum<file>, "error out"=w644:errorcluster)  [unwired: 1 in]
        n186 = Close File(refnum=w645, error in=w644) -> (error out=w636:errorcluster)  [unwired: 1 out]
      }
      frame "sample" {
        n187 = Number To Decimal String(number=w717) -> (decimal integer string=w716:string)  [unwired: 1 in]
        n188 = Fract/Exp String To Number(string=w713) -> (number=w673:dbl[])  [unwired: 3 in, 1 out]
        n189 = Concatenate Strings(w691, "-sample-" ("Substring"), w716, ".txt" ("Substring")) -> (w714:string)
        n190 = String To Path(string=w714) -> (path=w695:path)
        n191 = Index Array(array=w673, index=0 ("Index")) -> (element=w711:dbl)
        n192 = Index Array(array=w673, index=2 ("Index")) -> (element=w707:dbl)
        n193 = Index Array(array=w673, index=3 ("Index")) -> (element=w676:dbl)
        n194 = Index Array(array=w673, index=4 ("Index")) -> (element=w672:dbl)
        n195 = call <userlib>:"4155C Config Sampling Measurements.vi"("Sampling interval"=w672, "Sample time"=w676, "Display on/off"=TRUE, "Timings"=w682, "Num Points"=w707, "error in (no error)"=w719, "Drain Compliance"=w718, "Gate Compliance"=w692, "VISA session"=w720) -> ("error out"=w721:errorcluster, "dup VISA resource name"=w722:refnum<visa-resource-name>)  [unwired: 1 in]
        n196 = Index Array(array=w673, index=1 ("Index")) -> (element=w708:dbl)
        n197 = call <userlib>:"4155C Take Sample.vi"("Emergency Stop"=w688, "error in (no error)"=w721, "Vd"=w708, "Vg"=w711, "VISA resource name in"=w722) -> ("error out"=w686:errorcluster, "Id"=w724:dbl[], "Ig"=w697:dbl[], "VISA Resource Name out"=w684:refnum<visa-resource-name>, "Is"=w723:dbl[], "Time"=w701:dbl[])  [unwired: 1 in]
        n198 = Insert Into Array(array=dbl[][] [] ("Input Array"), new element=w701) -> (w700:dbl[][])  [unwired: 2 in]
        n199 = Insert Into Array(array=w700, new element=w697) -> (w699:dbl[][])  [unwired: 2 in]
        n200 = Insert Into Array(array=w699, new element=w724) -> (w698:dbl[][])  [unwired: 2 in]
        n201 = VISA Write(VISA resource name=w684, write buffer=":DISP ON" ("write buffer (\"\")"), error in (no error)=w686) -> (VISA resource name out=w683:refnum<visa-resource-name>, error out=w685:errorcluster)  [unwired: 1 out]
        n202 = Insert Into Array(array=w698, new element=w723) -> (w690:dbl[][])  [unwired: 2 in]
        n203 = Transpose 2D Array(2D array=w690) -> (transposed array=w689:dbl[][])
        n204 = call <vilib>:"compatOverwrite.vi"("overwrite (F)"=TRUE) -> ("overwrite?"=w670:T7)
        n205 = Open/Create/Replace File(file path (use dialog)=w695, error in=w685, operation (0:open)=w670) -> (refnum out=w704:refnum<file>, error out=w703:errorcluster)  [unwired: 3 in, 1 out]
        n206 = call <userlib>:"4155C Write array to file.vi"("Byte Stream File Refnum"=w704, "Header"=string[] ["Time /s", "Ig /A", "Id /A", "Is /A"], "Data Array"=w689, "error in (no error)"=w703) -> ("dup refnum"=w706:refnum<file>, "error out"=w705:errorcluster)  [unwired: 1 in]
        n207 = Close File(refnum=w706, error in=w705) -> (error out=w693:errorcluster)  [unwired: 1 out]
      }
      frame "samplei" {
        n208 = Number To Decimal String(number=w776) -> (decimal integer string=w775:string)  [unwired: 1 in]
        n209 = Fract/Exp String To Number(string=w772) -> (number=w738:dbl[])  [unwired: 3 in, 1 out]
        n210 = Concatenate Strings(w754, "-samplei-" ("Substring"), w775, ".txt" ("Substring")) -> (w773:string)
        n211 = String To Path(string=w773) -> (path=w757:path)
        n212 = Index Array(array=w738, index=4 ("Index")) -> (element=w732:dbl)
        n213 = Index Array(array=w738, index=3 ("Index")) -> (element=w733:dbl)
        n214 = Index Array(array=w738, index=1 ("Index")) -> (element=w735:dbl)
        n215 = Index Array(array=w738, index=0 ("Index")) -> (element=w736:dbl)
        n216 = Index Array(array=w738, index=2 ("Index")) -> (element=w734:dbl)
        n217 = call <userlib>:"4155C Config SamplingI Measurements.vi"("Sample time"=w734, "Display on/off"=TRUE, "Timings"=w746, "Num Points"=w735, "error in (no error)"=w778, "Sampling interval"=w733, "VISA session"=w779) -> ("error out"=w780:errorcluster, "dup VISA resource name"=w781:refnum<visa-resource-name>)  [unwired: 3 in]
        n218 = call <userlib>:"4155C Take SampleI.vi"("Emergency Stop"=w751, "error in (no error)"=w780, "Idg 2"=w736, "Vdg compliance 2"=w732, "VISA resource name in"=w781) -> ("error out"=w749:errorcluster, "Idg"=w783:dbl[], "Vdg"=w759:dbl[], "VISA Resource Name out"=w747:refnum<visa-resource-name>, "Is"=w782:dbl[], "Time"=w763:dbl[])  [unwired: 1 in]
        n219 = Insert Into Array(array=dbl[][] [] ("Input Array"), new element=w763) -> (w762:dbl[][])  [unwired: 2 in]
        n220 = Insert Into Array(array=w762, new element=w759) -> (w761:dbl[][])  [unwired: 2 in]
        n221 = Insert Into Array(array=w761, new element=w783) -> (w760:dbl[][])  [unwired: 2 in]
        n222 = VISA Write(VISA resource name=w747, write buffer=":DISP ON" ("write buffer (\"\")"), error in (no error)=w749) -> (VISA resource name out=w731:refnum<visa-resource-name>, error out=w748:errorcluster)  [unwired: 1 out]
        n223 = Insert Into Array(array=w760, new element=w782) -> (w753:dbl[][])  [unwired: 2 in]
        n224 = Transpose 2D Array(2D array=w753) -> (transposed array=w752:dbl[][])
        n225 = call <vilib>:"compatOverwrite.vi"("overwrite (F)"=TRUE) -> ("overwrite?"=w726:T7)
        n226 = Open/Create/Replace File(file path (use dialog)=w757, error in=w748, operation (0:open)=w726) -> (refnum out=w766:refnum<file>, error out=w765:errorcluster)  [unwired: 3 in, 1 out]
        n227 = call <userlib>:"4155C Write array to file.vi"("Byte Stream File Refnum"=w766, "Header"=string[] ["Time /s", "Vdg /V", "Idg /A", "Is /A"], "Data Array"=w752, "error in (no error)"=w765) -> ("dup refnum"=w768:refnum<file>, "error out"=w767:errorcluster)  [unwired: 1 in]
        n228 = Close File(refnum=w768, error in=w767) -> (error out=w729:errorcluster)  [unwired: 1 out]
        n229 = VISA Write(VISA resource name=w731, write buffer=";:PAGE:SCON:STAN OFF;:PAGE:CHAN:VSU2:DIS;" ("write buffer (\"\")"), error in (no error)=w729) -> (VISA resource name out=w727:refnum<visa-resource-name>, error out=w728:errorcluster)  [unwired: 1 out]
      }
      frame "#" {
        n230 = VISA Write(VISA resource name=w789, write buffer=":DISP ON" ("write buffer (\"\")"), error in (no error)=w788) -> (VISA resource name out=w787:refnum<visa-resource-name>, error out=w786:errorcluster)  [unwired: 1 out]
      }
      frame "stressV" {
        n231 = Number To Decimal String(number=w838) -> (decimal integer string=w837:string)  [unwired: 1 in]
        n232 = Fract/Exp String To Number(string=w834) -> (number=w806:dbl[])  [unwired: 3 in, 1 out]
        n233 = Concatenate Strings(w821, "-stressV-" ("Substring"), w837, ".txt" ("Substring")) -> (w835:string)
        n234 = String To Path(string=w835) -> (path=w825:path)
        n235 = Index Array(array=w806, index=3 ("Index")) -> (element=w803:dbl)
        n236 = Index Array(array=w806, index=1 ("Index")) -> (element=w801:dbl)
        n237 = Index Array(array=w806, index=0 ("Index")) -> (element=w800:dbl)
        n238 = Index Array(array=w806, index=4 ("Index")) -> (element=w805:dbl)
        n239 = Index Array(array=w806, index=2 ("Index")) -> (element=w802:dbl)
        n240 = call <userlib>:"4155C Config V Stress.vi"("VISA session"=w841, "ID compliance"=w803, "VD"=w801, "VG"=w800, "IG compliance"=w802, "error in (no error)"=w840, "Display on/off"=TRUE) -> ("dup VISA resource name"=w843:refnum<visa-resource-name>, "error out"=w842:errorcluster)
        n241 = call <userlib>:"4155C Apply Stress.vi"("error in (no error)"=w842, "Duration"=w805, "Emergency Stop"=w820, "VISA resource name in"=w843) -> ("error out"=w818:errorcluster, "VISA Resource Name out"=w816:refnum<visa-resource-name>)
        n242 = VISA Write(VISA resource name=w816, write buffer=":DISP ON" ("write buffer (\"\")"), error in (no error)=w818) -> (VISA resource name out=w815:refnum<visa-resource-name>, error out=w817:errorcluster)  [unwired: 1 out]
        n243 = call <vilib>:"compatOverwrite.vi"("overwrite (F)"=TRUE) -> ("overwrite?"=w799:T7)
        n244 = Open/Create/Replace File(file path (use dialog)=w825, error in=w817, operation (0:open)=w799) -> (refnum out=w828:refnum<file>, error out=w827:errorcluster)  [unwired: 3 in, 1 out]
        n245 = call <userlib>:"4155C Write array to file.vi"("Byte Stream File Refnum"=w828, "Header"=string[] ["V stress completed successfully", ""], "error in (no error)"=w827) -> ("dup refnum"=w830:refnum<file>, "error out"=w829:errorcluster)  [unwired: 2 in]
        n246 = Close File(refnum=w830, error in=w829) -> (error out=w823:errorcluster)  [unwired: 1 out]
      }
      frame "stressI" {
        n247 = Number To Decimal String(number=w880) -> (decimal integer string=w879:string)  [unwired: 1 in]
        n248 = Fract/Exp String To Number(string=w876) -> (number=w850:dbl[])  [unwired: 3 in, 1 out]
        n249 = Concatenate Strings(w863, "-stressI-" ("Substring"), w879, ".txt" ("Substring")) -> (w877:string)
        n250 = String To Path(string=w877) -> (path=w867:path)
        n251 = Index Array(array=w850, index=1 ("Index")) -> (element=w846:dbl)
        n252 = Index Array(array=w850, index=0 ("Index")) -> (element=w847:dbl)
        n253 = call <userlib>:"4155C Config I Stress.vi"("VISA session"=w883, "IDG"=w847, "VDG compliance"=w846, "error in (no error)"=w882, "Display on/off"=TRUE) -> ("dup VISA resource name"=w885:refnum<visa-resource-name>, "error out"=w884:errorcluster)
        n254 = Index Array(array=w850, index=2 ("Index")) -> (element=w848:dbl)
        n255 = call <userlib>:"4155C Apply Stress.vi"("error in (no error)"=w884, "Duration"=w848, "Emergency Stop"=w862, "VISA resource name in"=w885) -> ("error out"=w860:errorcluster, "VISA Resource Name out"=w858:refnum<visa-resource-name>)
        n256 = VISA Write(VISA resource name=w858, write buffer=":DISP ON" ("write buffer (\"\")"), error in (no error)=w860) -> (VISA resource name out=w857:refnum<visa-resource-name>, error out=w859:errorcluster)  [unwired: 1 out]
        n257 = call <vilib>:"compatOverwrite.vi"("overwrite (F)"=TRUE) -> ("overwrite?"=w845:T7)
        n258 = Open/Create/Replace File(file path (use dialog)=w867, error in=w859, operation (0:open)=w845) -> (refnum out=w870:refnum<file>, error out=w869:errorcluster)  [unwired: 3 in, 1 out]
        n259 = call <userlib>:"4155C Write array to file.vi"("Byte Stream File Refnum"=w870, "Header"=string[] ["I stress completed successfully", ""], "error in (no error)"=w869) -> ("dup refnum"=w872:refnum<file>, "error out"=w871:errorcluster)  [unwired: 2 in]
        n260 = Close File(refnum=w872, error in=w871) -> (error out=w865:errorcluster)  [unwired: 1 out]
      }
      frame "vsu2pulse" {
        n261 = Number To Decimal String(number=w920) -> (decimal integer string=w919:string)  [unwired: 1 in]
        n262 = Fract/Exp String To Number(string=w916) -> (number=w891:dbl[])  [unwired: 3 in, 1 out]
        n263 = Concatenate Strings(w904, "-vsu2-" ("Substring"), w919, ".txt" ("Substring")) -> (w917:string)
        n264 = String To Path(string=w917) -> (path=w908:path)
        n265 = Index Array(array=w891, index=1 ("Index")) -> (element=w890:dbl)
        n266 = Index Array(array=w891, index=0 ("Index")) -> (element=w888:dbl)
        n267 = call <userlib>:"4155C Config VSU2 Stress.vi"("error in (no error)"=w922, "VSU2"=w888, "Display on/off"=TRUE, "VISA session"=w923) -> ("error out"=w924:errorcluster, "dup VISA resource name"=w925:refnum<visa-resource-name>)
        n268 = call <userlib>:"4155C Apply Stress.vi"("error in (no error)"=w924, "Duration"=w890, "Emergency Stop"=w903, "VISA resource name in"=w925) -> ("error out"=w901:errorcluster, "VISA Resource Name out"=w899:refnum<visa-resource-name>)
        n269 = VISA Write(VISA resource name=w899, write buffer=":DISP ON" ("write buffer (\"\")"), error in (no error)=w901) -> (VISA resource name out=w898:refnum<visa-resource-name>, error out=w900:errorcluster)  [unwired: 1 out]
        n270 = call <vilib>:"compatOverwrite.vi"("overwrite (F)"=TRUE) -> ("overwrite?"=w887:T7)
        n271 = Open/Create/Replace File(file path (use dialog)=w908, error in=w900, operation (0:open)=w887) -> (refnum out=w911:refnum<file>, error out=w910:errorcluster)  [unwired: 3 in, 1 out]
        n272 = call <userlib>:"4155C Write array to file.vi"("Byte Stream File Refnum"=w911, "Header"=string[] ["VSU2 pulse completed successfully", ""], "error in (no error)"=w910) -> ("dup refnum"=w913:refnum<file>, "error out"=w912:errorcluster)  [unwired: 2 in]
        n273 = Close File(refnum=w913, error in=w912) -> (error out=w906:errorcluster)  [unwired: 1 out]
      }
      frame "sample-fpp" {
        w934 = string[] ["Time /s", "Id VgVd /A", "Ig VgVd /A", "Vp1 VgVd /V", "Vp2 VgVd /V"] ("Header")
        w938 = "%d" ("format string")
        n274 = Number To Decimal String(number=w988) -> (decimal integer string=w987:string)  [unwired: 1 in]
        n275 = Fract/Exp String To Number(string=w984) -> (number=w972:dbl[])  [unwired: 3 in, 1 out]
        n276 = Concatenate Strings(w978, "-samplefpp-" ("Substring"), w987, ".txt" ("Substring")) -> (w985:string)
        n277 = String To Path(string=w985) -> (path=w946:path)
        n278 = Index Array(array=w972, index=0 ("Index")) -> (element=w932:dbl)
        n279 = Index Array(array=w972, index=1 ("Index")) -> (element=w931:dbl)
        n280 = Index Array(array=w972, index=2 ("Index")) -> (element=w980:dbl)
        n281 = Index Array(array=w972, index=3 ("Index")) -> (element=w970:dbl)
        n282 = call <userlib>:"4155C Config Sampling Measurements FPP.vi"("VISA session"=w991, "Num Points"=w980, "Vg"=w932, "Display on/off"=TRUE, "Gate Compliance"=w979, "Drain Compliance"=w989, "Standby"="Standby", "error in (no error)"=w990, "Timings"=w977, "Vd"=w931, "Sample time"=w970) -> ("dup VISA resource name"=w948:refnum<visa-resource-name>, "error out"=w947:errorcluster)  [unwired: 3 in]
        n283 = Number To Decimal String(number=w932) -> (decimal integer string=w958:string)  [unwired: 1 in]
        n284 = call <userlib>:"4155C Take Sample FPP.vi"("VISA resource name in"=w948, "error in (no error)"=w947, "Emergency Stop"=w949) -> ("Time"=w953:dbl[], "Vp1"=w963:dbl[], "VISA Resource Name out"=w929:refnum<visa-resource-name>, "Ig"=w951:dbl[], "Id"=w952:dbl[], "Vp2"=w961:dbl[], "error out"=w950:errorcluster)  [unwired: 10 in]
        n285 = Insert Into Array(array=dbl[][] [] ("Input Array"), new element=w953) -> (w967:dbl[][])  [unwired: 2 in]
        n286 = Number To Decimal String(number=w931) -> (decimal integer string=w956:string)  [unwired: 1 in]
        n287 = Insert Into Array(array=w967, new element=w952) -> (w966:dbl[][])  [unwired: 2 in]
        n288 = Concatenate Strings("(Vg = " ("Substring"), w958, "V, Vd = " ("Substring"), w956, "V)" ("Substring")) -> (w954:string)
        n289 = Insert Into Array(array=w966, new element=w951) -> (w965:dbl[][])  [unwired: 2 in]
        n290 = Insert Into Array(array=w965, new element=w963) -> (w962:dbl[][])  [unwired: 2 in]
        n291 = Insert Into Array(array=w962, new element=w961) -> (w930:dbl[][])  [unwired: 2 in]
        n292 = call <vilib>:"compatOverwrite.vi"("overwrite (F)"=TRUE) -> ("overwrite?"=w927:T7)
        n293 = Open/Create/Replace File(file path (use dialog)=w946, error in=w950, operation (0:open)=w927) -> (refnum out=w943:refnum<file>, error out=w944:errorcluster)  [unwired: 3 in, 1 out]
        n294 = Array To Spreadsheet String(array=w934, 3:w938) -> (spreadsheet string=w940:string)  [unwired: 1 in]
        n295 = Transpose 2D Array(2D array=w930) -> (transposed array=w960:dbl[][])
        n296 = Search and Replace String(replace all?=TRUE ("replace all? (F)"), input string=w940, search string="VgVd", replace string=w954) -> (result string=w936:string)  [unwired: 4 in, 3 out]
        n297 = Spreadsheet String To Array(format string=w938, spreadsheet string=w936, array type (2D Dbl)=w934) -> (array=w935:string[])  [unwired: 1 in]
        n298 = call <userlib>:"4155C Write array to file.vi"("Byte Stream File Refnum"=w943, "Header"=w935, "Data Array"=w960, "error in (no error)"=w944) -> ("dup refnum"=w941:refnum<file>, "error out"=w942:errorcluster)  [unwired: 1 in]
        n299 = Close File(refnum=w941, error in=w942) -> (error out=w928:errorcluster)  [unwired: 1 out]
      }
      frame "resample-fpp" {
        w1002 = string[] ["Time /s", "Id VgVd /A", "Ig VgVd /A", "Vp1 VgVd /V", "Vp2 VgVd /V"] ("Header")
        w1006 = "%d" ("format string")
        n300 = Number To Decimal String(number=w1048) -> (decimal integer string=w1047:string)  [unwired: 1 in]
        n301 = Fract/Exp String To Number(string=w1044) -> (number=w995:dbl[])  [unwired: 3 in, 1 out]
        n302 = Concatenate Strings(w1040, "-resamplefpp-" ("Substring"), w1047, ".txt" ("Substring")) -> (w1045:string)
        n303 = String To Path(string=w1045) -> (path=w1014:path)
        n304 = Index Array(array=w995, index=0 ("Index")) -> (element=w1001:dbl)
        n305 = Index Array(array=w995, index=1 ("Index")) -> (element=w1000:dbl)
        n306 = Number To Decimal String(number=w1001) -> (decimal integer string=w1024:string)  [unwired: 1 in]
        n307 = call <userlib>:"4155C Take Sample FPP.vi"("VISA resource name in"=w997, "error in (no error)"=w996, "Emergency Stop"=w1015) -> ("Time"=w1019:dbl[], "Vp1"=w1029:dbl[], "VISA Resource Name out"=w999:refnum<visa-resource-name>, "Ig"=w1017:dbl[], "Id"=w1018:dbl[], "Vp2"=w1027:dbl[], "error out"=w1016:errorcluster)  [unwired: 10 in]
        n308 = Insert Into Array(array=dbl[][] [] ("Input Array"), new element=w1019) -> (w1033:dbl[][])  [unwired: 2 in]
        n309 = Number To Decimal String(number=w1000) -> (decimal integer string=w1022:string)  [unwired: 1 in]
        n310 = Insert Into Array(array=w1033, new element=w1018) -> (w1032:dbl[][])  [unwired: 2 in]
        n311 = Concatenate Strings("(Vg = " ("Substring"), w1024, "V, Vd = " ("Substring"), w1022, "V)" ("Substring")) -> (w1020:string)
        n312 = Insert Into Array(array=w1032, new element=w1017) -> (w1031:dbl[][])  [unwired: 2 in]
        n313 = Insert Into Array(array=w1031, new element=w1029) -> (w1028:dbl[][])  [unwired: 2 in]
        n314 = Insert Into Array(array=w1028, new element=w1027) -> (w994:dbl[][])  [unwired: 2 in]
        n315 = call <vilib>:"compatOverwrite.vi"("overwrite (F)"=TRUE) -> ("overwrite?"=w993:T7)
        n316 = Open/Create/Replace File(file path (use dialog)=w1014, error in=w1016, operation (0:open)=w993) -> (refnum out=w1011:refnum<file>, error out=w1012:errorcluster)  [unwired: 3 in, 1 out]
        n317 = Array To Spreadsheet String(array=w1002, 3:w1006) -> (spreadsheet string=w1008:string)  [unwired: 1 in]
        n318 = Transpose 2D Array(2D array=w994) -> (transposed array=w1026:dbl[][])
        n319 = Search and Replace String(replace all?=TRUE ("replace all? (F)"), input string=w1008, search string="VgVd", replace string=w1020) -> (result string=w1004:string)  [unwired: 4 in, 3 out]
        n320 = Spreadsheet String To Array(format string=w1006, spreadsheet string=w1004, array type (2D Dbl)=w1002) -> (array=w1003:string[])  [unwired: 1 in]
        n321 = call <userlib>:"4155C Write array to file.vi"("Byte Stream File Refnum"=w1011, "Header"=w1003, "Data Array"=w1026, "error in (no error)"=w1012) -> ("dup refnum"=w1009:refnum<file>, "error out"=w1010:errorcluster)  [unwired: 1 in]
        n322 = Close File(refnum=w1009, error in=w1010) -> (error out=w998:errorcluster)  [unwired: 1 out]
      }
    }
    n323 = local write "Lines left to run:"(w43) -> ()
    n324 = Empty String/Path?(string/path=w43) -> (empty?=w79:bool)
    n325 = Not(x=w79) -> (.not. x?=w78:bool)
  }
